vi "Measurment.vi"() -> ()   [LabVIEW 2015]
panel:
  out "Waveform Chart":dbl(graph)
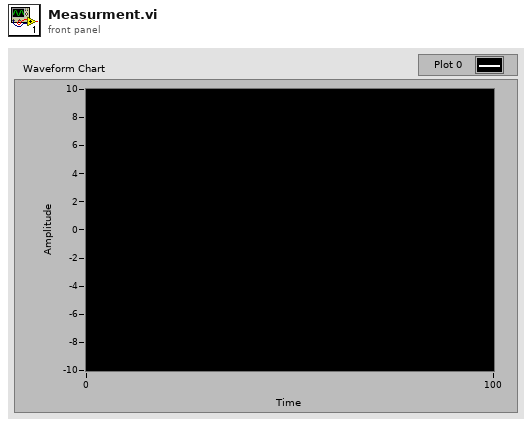
[diagram p1: front panel]
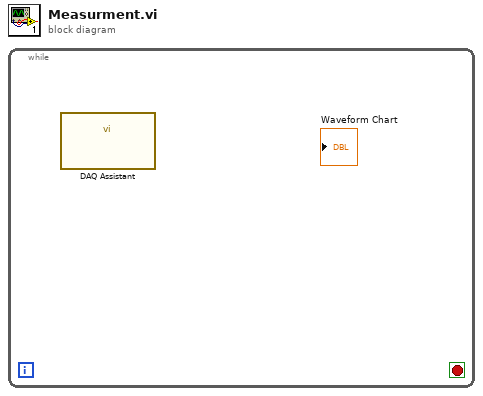
[diagram p0: block diagram]
diagram:
  n1 = while {
    stop <- _ stop-if-true
    n2 = call "DAQ Assistant"() -> ()  [unwired: 12 in]
  }
